vi "Conditionally Save Temporary System Definition.vi"(8 "error in (no error)":errorcluster, 10 "Save?":bool, 11 "Test Case":refnum<class "SLSC Switch Scripting Unit Tests.lvclass">) -> (0 "error out":errorcluster, 2 "filename":string, 3 "Test Case":refnum<class "SLSC Switch Scripting Unit Tests.lvclass">)   [LabVIEW 2019, in "SLSC Switch Scripting Unit Tests.lvclass"]
uses:
  SLSC Switch Scripting Unit Tests.lvclass
  SLSC Switch Scripting Unit Tests.lvclass/SLSC Switch Scripting Unit Tests.ctl
  NationalInstruments.VeriStand.SystemDefinitionAPI
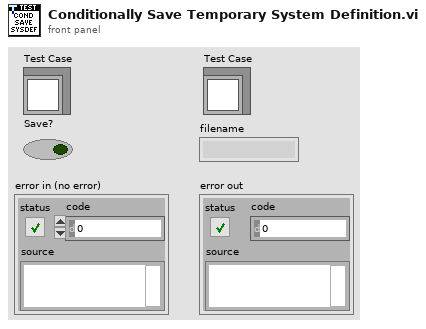
[diagram p1: front panel]
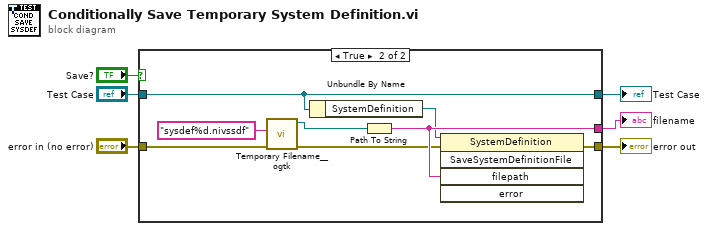
[diagram p0: block diagram]
diagram:
  n1 = case shown="True" "Save?" {
    tunnel: "error in (no error)" -> [w8 w16]
    tunnel: [_ w15] -> w5
    tunnel: [w8 w11] -> w4
    tunnel: "Test Case" -> [w7 w9]
    tunnel: [w7 w9] -> w1
    frame False {
    }
    frame True {
      n2 = call <userlib>:"Temporary Filename__ogtk.vi"("error in (no error)"=w16, "pattern (lvtemp%d.tmp)"="sysdef%d.nivssdf") -> ("error out"=w14:errorcluster, "file in tmp dir"=w13:path)  [unwired: 4 in]
      n3 = Unbundle By Name(w9) -> ("SystemDefinition"=w10:refnum<k24>)
      n4 = Path To String(path=w13) -> (string=w15:string)
      n5 = invoke class="SystemDefinition" method="SaveSystemDefinitionFile"(reference=w10, error in=w14, "filepath"=w15) -> (error out=w11:errorcluster)  [unwired: 2 in, 4 out]
    }
  }
  "filename" <- w5
  "error out" <- w4
  "Test Case" <- w1
